vi "Page Template.vi"() -> ()   [LabVIEW 2018]
uses:
  <vilib>/NI/STM/TCP/Read Meta Data (TCP Ref).vi
  <vilib>/NI/STM/TCP/Get Connection Reference (TCP).vi
  <vilib>/NI/AMC/Read Termination Message.vi
  <vilib>/NI/AMC/Create Single Message.vi
  <vilib>/NI/AMC/Update Message Routing Info.vi
  <vilib>/NI/STM/TCP/Read Meta Data (TCP Clst).vi
  <vilib>/NI/AMC/Globals.vi
  <vilib>/NI/STM/TCP/Write Message (TCP).vi
  <vilib>/NI/AMC/Send Message.vi
  <vilib>/NI/AMC/AMC.lvlib
  <vilib>/NI/STM/NI STM.lvlib
panel:
  out "Run Enabled":bool
  in  "Dosing":bool
  in  "Mixing Tank":bool
  in  "Process 3":bool
  in  "Process 2":bool
  in  "Process 1":bool
  out "status":string
  in  "Home Btn":bool
  in  "Facilities Btn":bool
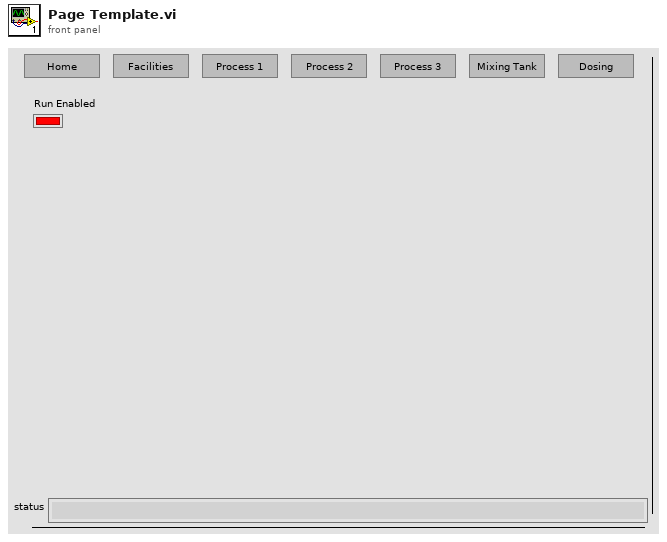
[diagram p1: front panel]
types:
  T1 = typedef "AMC.lvlib/Message Queue.ctl" = refnum<queue>
  T2 = typedef "NI STM.lvlib/TCP Connection Info.ctl" = cluster{"connection ID":refnum<k5>, "meta data":T3[]}
  T3 = typedef "NI STM.lvlib/MetaDataElement.ctl" = string
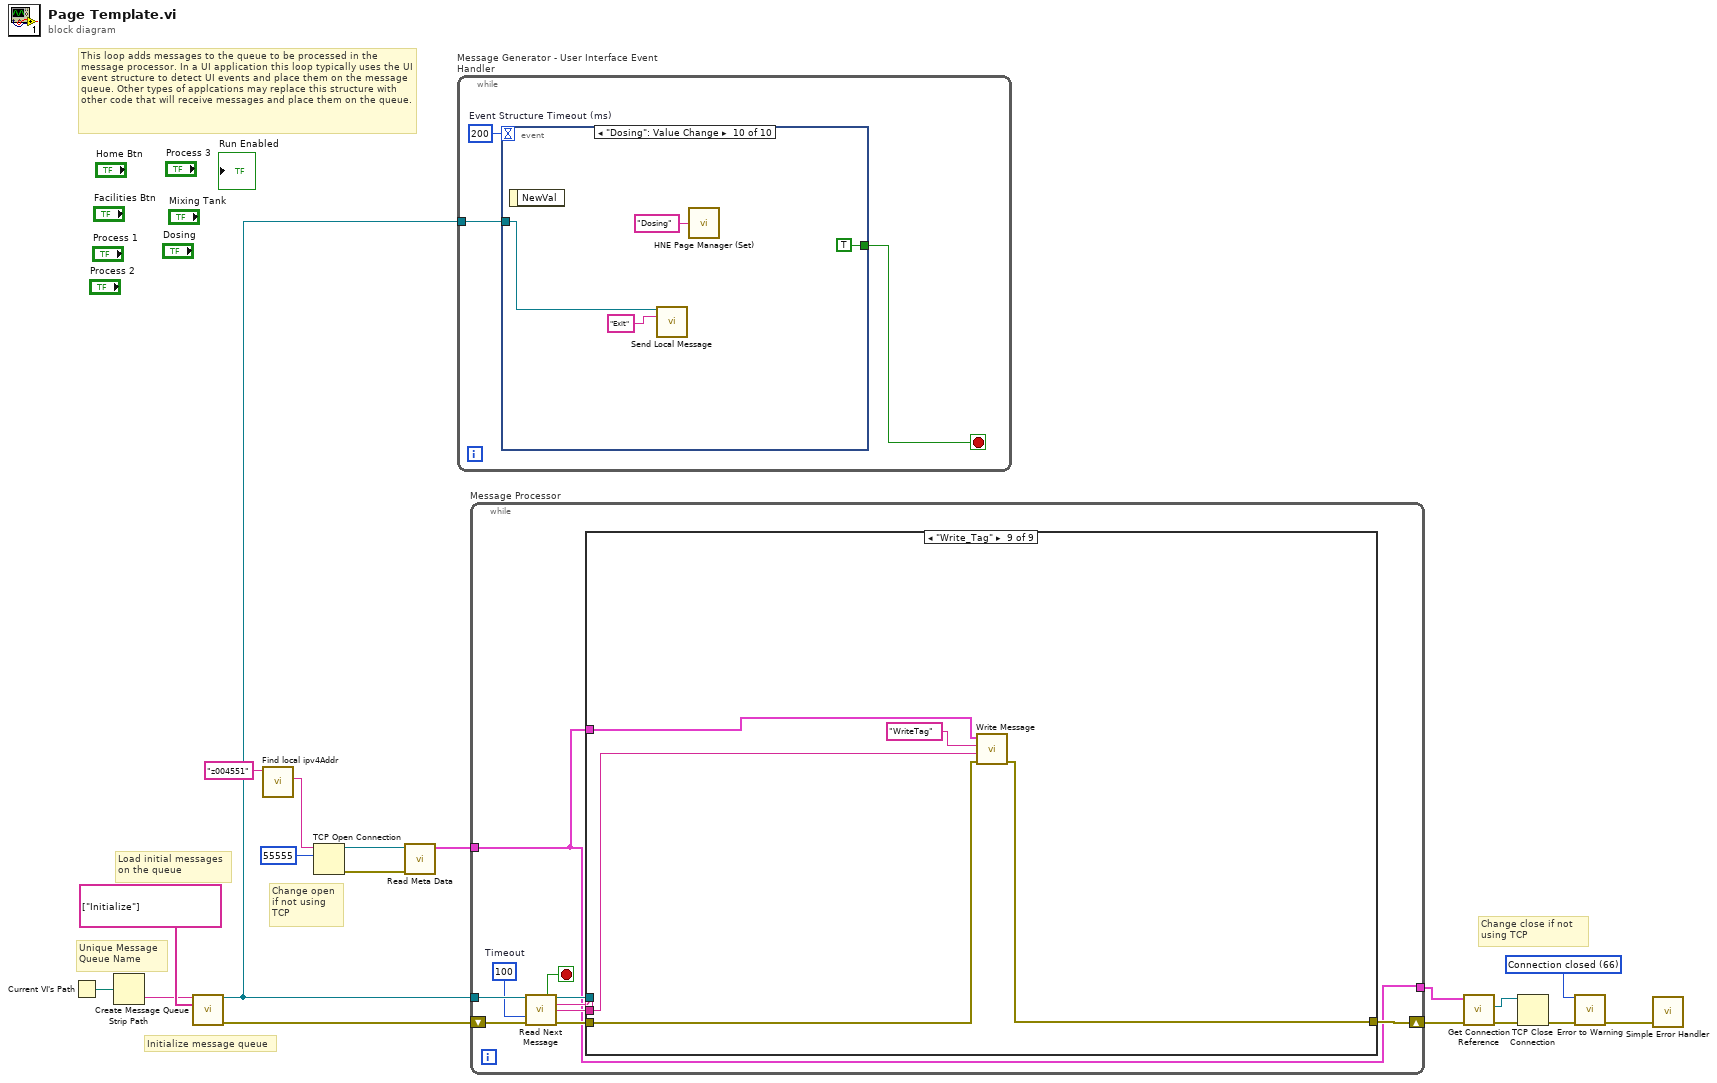
[diagram p0: block diagram]
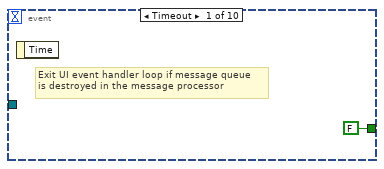
[diagram p2: hidden frame]
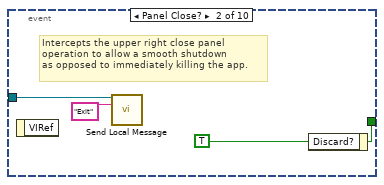
[diagram p3: hidden frame]
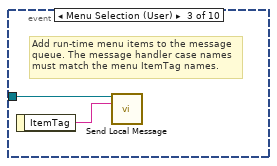
[diagram p4: hidden frame]
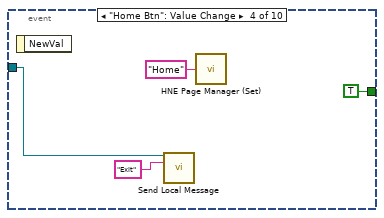
[diagram p5: hidden frame]
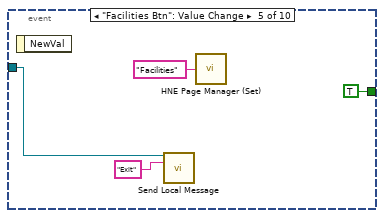
[diagram p6: hidden frame]
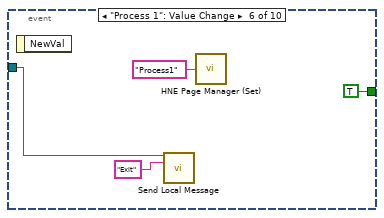
[diagram p7: hidden frame]
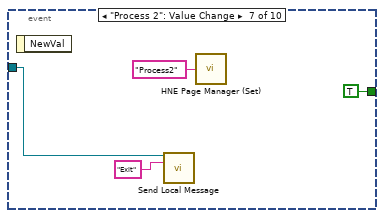
[diagram p8: hidden frame]
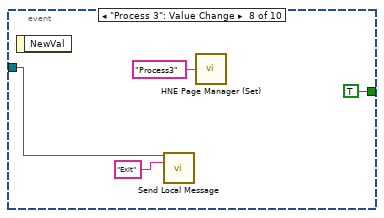
[diagram p9: hidden frame]
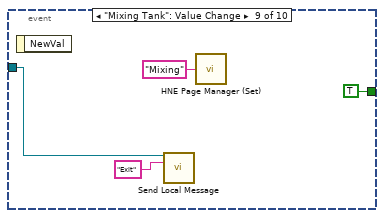
[diagram p10: hidden frame]
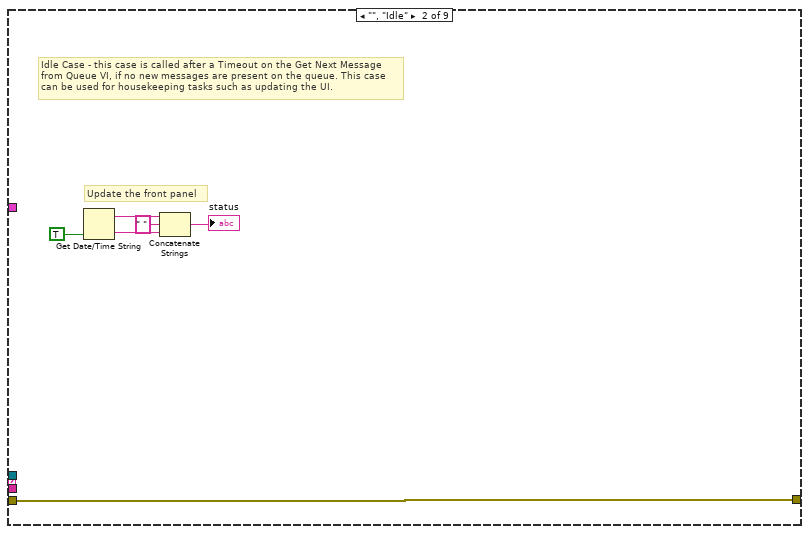
[diagram p12: hidden frame]
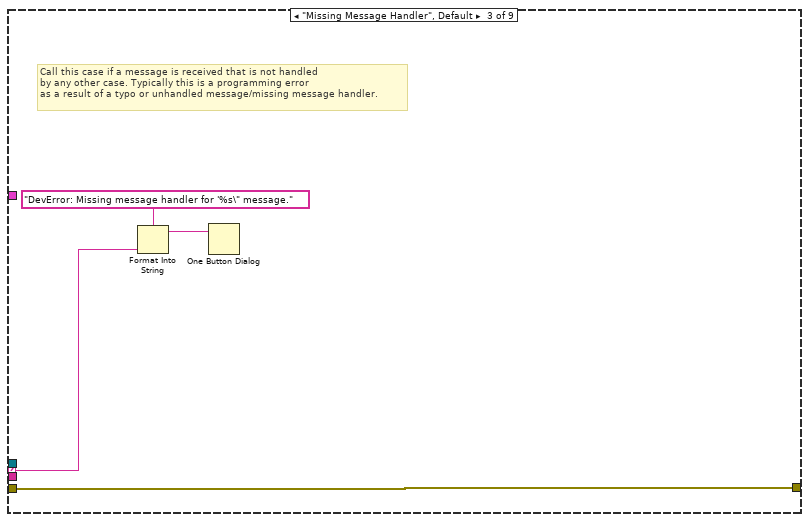
[diagram p13: hidden frame]
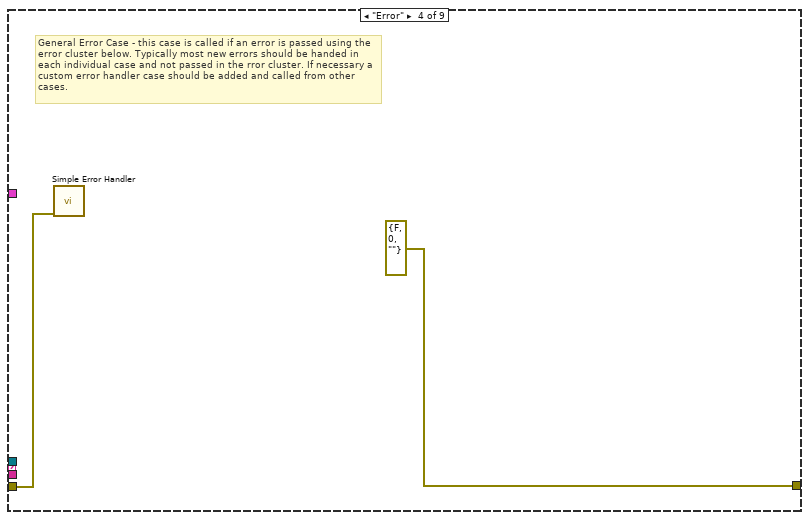
[diagram p14: hidden frame]
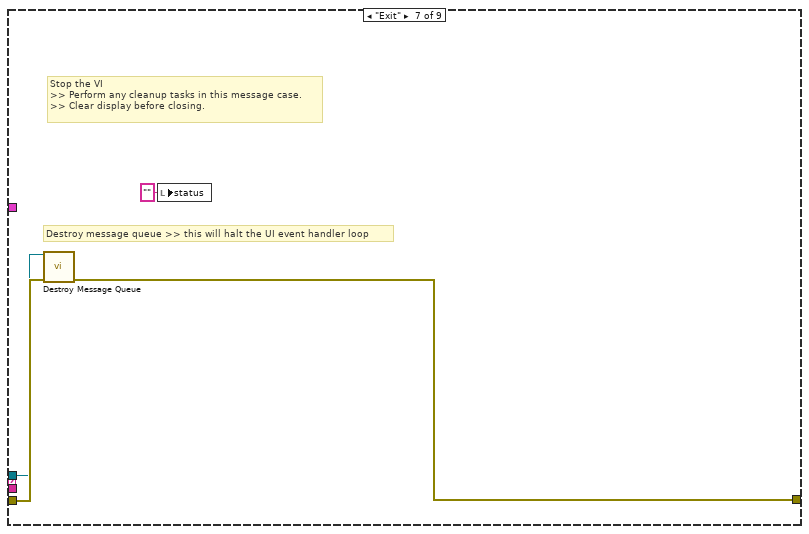
[diagram p17: hidden frame]
diagram:
  w7 = 66 items=["No Error", "Argument Error", "Memory Full", "Out of Zone", "End of File", "File Already Open", "Generic File IO Error", "File Not Found", "File Permission Error", "Disk Full", "Duplicate Path", "Too Many Files Open", "Not Enabled", "Resource File Not Found", "Cannot Add Resource", "Resource Not Found", "Image Not Found", "Image Memory Error", "Pen Does Not Exist", "Config Bad Type", "Config Token Not Found", "Config Parse Error", "Config Memory Error", "Bad External Code Format", "Bad External Code Offset", "External Code Not Present", "Null Window", "Destroy Window Mixup", "Null Menu", "Print Aborted", "Bad Print Record", "Print Driver Error", "Windows Error During Print", "Memory Error During Print", "Print Dialog Error", "Generic Print Error", "Invalid Device Refnum", "Device Not Found", "Device Parameter Error", "Device Unit Error", "Can't Open Device", "Device Call Aborted", "Generic Error", "Cancelled By User", "Object ID Too Low", "Object ID Too High", "Object Not In Heap", "Unknown Heap", "Bad DefProc ID", "DefProc Not In Table", "Message Out Of Range", "Null Method", "Unknown Message", "Manager Call Not Supported", "Bad address", "Connection In progress", "Connection timed out", "Connection is already in progress", "Network attribute not supported", "Network error", "Address in use", "System out of memory", "Connection aborted", "Connection refused", "Connection is not connected", "Connection is already connected", "Connection closed", "Initialize error (interapplication manager)", "Bad occurrence", "Wait on unbound occurrence handler", "Occurrence queue overflow", "Bad path", "Semaphore not signaled", "Unrecognized type (interapplication manager)"] ("1st Error to Convert")
  # "Change close if not using TCP"
  # "Change open if not using TCP"
  # "This loop adds messages to the queue to be processed in the message processor. In a UI application this loop typically uses the UI event structure to detect UI events and place them on the message queue. Other types of applcations may replace this structure with other code that will receive messages and place them on the queue."
  # "Initialize message queue"
  # "Unique Message\nQueue Name"
  # "Load initial messages\non the queue"
  n1 = Current VI's Path() -> (path=w14:path)
  n2 = Strip Path(path=w14) -> (name=w17:string)  [unwired: 1 out]
  n3 = call <vilib>:"Create Message Queue.vi"("message queue name"=w17, "initial message names"=string[] ["Initialize"]) -> ("message queue out"=w16:T1, "error out"=w15:errorcluster)  [unwired: 12 in]
  n4 = call "Find local ipv4Addr.vi"("MachineToFind"="z004551") -> ("name"=w10:string)  [unwired: 9 in, 1 out]
  n5 = TCP Open Connection(address=w10, remote port or service name=u16 55555 ("remote port")) -> (connection ID=w12:refnum<k5>, error out=w11:errorcluster)  [unwired: 1 in, 2 out]
  n6 = call-poly <vilib>:"Read Meta Data.vi"("error in"=w11, "connection ID"=w12) -> ("connection info out"=w2:T2)  [unwired: 7 in, 2 out]
  n7 = while "Message Generator - User Interface Event Handler" {
    tunnel: w16 -> [w19]
    stop <- w20 stop-if-true
    w21 = 200  # Event Structure Timeout (ms)
    n8 = event shown="[9] \"Dosing\": Value Change" {
      selector: _ -> [_ _ _ _ _ _ _ _ _ _]
      dyn-events: _ -> [_ _ _ _ _ _ _ _ _ _]
      timeout: w21 -> [_ _ _ _ _ _ _ _ _ _]
      tunnel: [FALSE ("Discard?") w25 _ TRUE ("Discard?") TRUE ("Discard?") TRUE ("Discard?") TRUE ("Discard?") TRUE ("Discard?") TRUE ("Discard?") TRUE ("Discard?")] -> w20
      tunnel: w19 -> [_ w23 w26 w28 w32 w36 w40 w44 w48 w52]
      event Timeout {
        # "Exit UI event handler loop if message queue\nis destroyed in the message processor"
        n9 = event-data() -> ()  [unwired: 2 out]
      }
      event Panel Close? {
        w25 = TRUE ("Discard?")
        # "Intercepts the upper right close panel\noperation to allow a smooth shutdown\nas opposed to immediately killing the app."
        n10 = event-data() -> ()  [unwired: 2 out]
        n11 = call <vilib>:"Send Local Message.vi"("message queue in"=w23, "message name"="Exit") -> ()  [unwired: 11 in, 3 out]
        n12 = event-data("Discard?"=w25) -> ()  [unwired: 1 in, 1 out]
      }
      event Menu Selection (User) {
        # "Add run-time menu items to the message\nqueue. The message handler case names must match the menu ItemTag names."
        n13 = event-data() -> ("ItemTag"=w27:string)  [unwired: 1 out]
        n14 = call <vilib>:"Send Local Message.vi"("message queue in"=w26, "message name"=w27) -> ()  [unwired: 11 in, 3 out]
      }
      event "Home Btn": Value Change {
        n15 = event-data() -> ()  [unwired: 2 out]
        n16 = call <vilib>:"Send Local Message.vi"("message queue in"=w28, "message name"="Exit") -> ()  [unwired: 11 in, 3 out]
        n17 = call <userlib>:"HNE Page Manager (Set).vi"("Next Page"="Home") -> ()  [unwired: 4 in, 1 out]
      }
      event "Facilities Btn": Value Change {
        n18 = event-data() -> ()  [unwired: 2 out]
        n19 = call <vilib>:"Send Local Message.vi"("message queue in"=w32, "message name"="Exit") -> ()  [unwired: 11 in, 3 out]
        n20 = call <userlib>:"HNE Page Manager (Set).vi"("Next Page"="Facilities") -> ()  [unwired: 4 in, 1 out]
      }
      event "Process 1": Value Change {
        n21 = event-data() -> ()  [unwired: 2 out]
        n22 = call <vilib>:"Send Local Message.vi"("message queue in"=w36, "message name"="Exit") -> ()  [unwired: 11 in, 3 out]
        n23 = call <userlib>:"HNE Page Manager (Set).vi"("Next Page"="Process1") -> ()  [unwired: 4 in, 1 out]
      }
      event "Process 2": Value Change {
        n24 = event-data() -> ()  [unwired: 2 out]
        n25 = call <vilib>:"Send Local Message.vi"("message queue in"=w40, "message name"="Exit") -> ()  [unwired: 11 in, 3 out]
        n26 = call <userlib>:"HNE Page Manager (Set).vi"("Next Page"="Process2") -> ()  [unwired: 4 in, 1 out]
      }
      event "Process 3": Value Change {
        n27 = event-data() -> ()  [unwired: 2 out]
        n28 = call <vilib>:"Send Local Message.vi"("message queue in"=w44, "message name"="Exit") -> ()  [unwired: 11 in, 3 out]
        n29 = call <userlib>:"HNE Page Manager (Set).vi"("Next Page"="Process3") -> ()  [unwired: 4 in, 1 out]
      }
      event "Mixing Tank": Value Change {
        n30 = event-data() -> ()  [unwired: 2 out]
        n31 = call <vilib>:"Send Local Message.vi"("message queue in"=w48, "message name"="Exit") -> ()  [unwired: 11 in, 3 out]
        n32 = call <userlib>:"HNE Page Manager (Set).vi"("Next Page"="Mixing") -> ()  [unwired: 4 in, 1 out]
      }
      event "Dosing": Value Change {
        n33 = event-data() -> ()  [unwired: 2 out]
        n34 = call <vilib>:"Send Local Message.vi"("message queue in"=w52, "message name"="Exit") -> ()  [unwired: 11 in, 3 out]
        n35 = call <userlib>:"HNE Page Manager (Set).vi"("Next Page"="Dosing") -> ()  [unwired: 4 in, 1 out]
      }
    }
  }
  n36 = while "Message Processor" {
    shift-left: w15 -> [w61]
    shift-right: [w65] -> w3
    tunnel: w16 -> [w62]
    tunnel: [w56] -> w1
    tunnel: w2 -> [w56]
    stop <- w64 stop-if-true
    w57 = 100  # Timeout
    n37 = call <vilib>:"Read Next Message.vi"("message queue in"=w62, "timeout (1 ms)"=w57, "error in"=w61) -> ("exit process?"=w64:bool, "message queue out"=w63:T1, "message name"=w59:string, "message value"=w58:string, "error out"=w60:errorcluster)  [unwired: 5 in, 3 out]
    n38 = case shown="\"Write_Tag\"" w59 {
      selector: w59 -> [_ _ w75 _ _ _ _ _ _]
      tunnel: w63 -> [_ _ _ _ _ _ w82 _ _]
      tunnel: w60 -> [w66 w72 w76 w77 w79 w80 w83 w85 w87]
      tunnel: [w66 w72 w76 errorcluster {"status"=FALSE, "code"=0, "source"=""} ("error out") w79 w80 w81 w85 w86] -> w65
      tunnel: w58 -> [_ _ _ _ _ _ _ _ w88]
      tunnel: w56 -> [_ _ _ _ _ _ _ _ w89]
      frame "---------- Framework Operations ----------" {
        # "Dummy case to add a seperator in the Case Structure menu"
      }
      frame "", "Idle" {
        # "Update the front panel"
        # "Idle Case - this case is called after a Timeout on the Get Next Message from Queue VI, if no new messages are present on the queue. This case can be used for housekeeping tasks such as updating the UI."
        n39 = Get Date/Time String(want seconds? (F)=TRUE) -> (date string=w71:string, time string=w70:string)  [unwired: 2 out]
        n40 = Concatenate Strings(w71, " " ("string"), w70) -> (→"status":string)
      }
      frame "Missing Message Handler", Default {
        # "Call this case if a message is received that is not handled \nby any other case. Typically this is a programming error\nas a result of a typo or unhandled message/missing message handler."
        n41 = Format Into String(format string="DevError: Missing message handler for '%s\" message." ("message"), w75) -> (resulting string=w73:string)  [unwired: 2 in, 1 out]
        n42 = One Button Dialog(message=w73) -> ()  [unwired: 2 out]
      }
      frame "Error" {
        # "General Error Case - this case is called if an error is passed using the error cluster below. Typically most new errors should be handed in each individual case and not passed in the rror cluster. If necessary a custom error handler case should be added and called from other cases."
        n43 = call <vilib>:"Simple Error Handler.vi"("error in (no error)"=w77) -> ()  [unwired: 1 in, 8 out]
      }
      frame "---------- Generic Operations ----------" {
        # "Dummy case to add a seperator in the Case Structure menu"
      }
      frame "Initialize" {
        # "Initialize the state variables and user interface"
      }
      frame "Exit" {
        # "Destroy message queue >> this will halt the UI event handler loop"
        # "Stop the VI\n>> Perform any cleanup tasks in this message case.\n>> Clear display before closing."
        n44 = call <vilib>:"Destroy Message Queue.vi"("message queue in"=w82, "error in"=w83) -> ("error out"=w81:errorcluster)  [unwired: 11 in, 2 out]
        n45 = local write "status"("" ("Status")) -> ()
      }
      frame "---------- Application Operations ----------" {
        # "Dummy case to add a seperator in the Case Structure menu"
      }
      frame "Write_Tag" {
        n46 = call-poly <vilib>:"Write Message.vi"("error in"=w87, "data"=w88, "name"="WriteTag", "connection info in"=w89) -> ("error out"=w86:errorcluster)  [unwired: 6 in, 1 out]
      }
    }
  }
  n47 = call-poly <vilib>:"Get Connection Reference.vi"("error in"=w3, "connection info in"=w1) -> ("error out"=w6:errorcluster, "connection ID out"=w5:refnum<k5>)  [unwired: 8 out]
  n48 = TCP Close Connection(connection ID=w5, error in (no error)=w6) -> (error out=w8:errorcluster)  [unwired: 2 out]
  n49 = call <vilib>:"Error to Warning.vi"("1st Error to Convert"=w7, "error in"=w8) -> ("warning out"=w4:errorcluster)  [unwired: 3 in, 10 out]
  n50 = call <vilib>:"Simple Error Handler.vi"("error in (no error)"=w4) -> ()  [unwired: 4 in, 5 out]
